vi "Load App.vi"(8 "error in (no error)":errorcluster, 11 "Status Notifier":refnum<notifier>) -> (0 "error out":errorcluster)   [LabVIEW 2012, in "Car Wash Controller.lvlib" / "Car Wash Controller.lvclass"]
doc: "Load the application into memory and start it running. The input notifier is used to send text to the splash screen to tell the user what stage the load process is in."
uses:
  Car Wash Controller.lvclass
  <vilib>/ActorFramework/Message Queue/Message Queue.lvclass/Message Queue.ctl
  <vilib>/ActorFramework/Actor/Actor.lvclass
  <vilib>/ActorFramework/Message Queue/Message Queue.lvclass
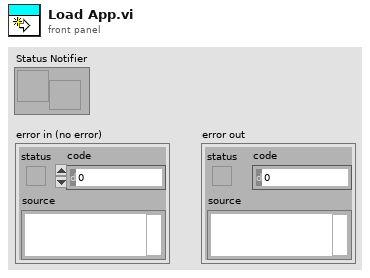
[diagram p1: front panel]
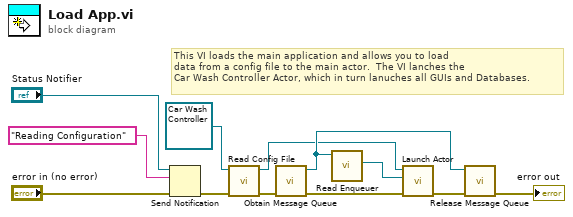
[diagram p0: block diagram]
diagram:
  # "This VI loads the main application and allows you to load\ndata from a config file to the main actor.  The VI lanches the\nCar Wash Controller Actor, which in turn lanuches all GUIs and Databases."
  n1 = Send Notification(notification="Reading Configuration", notifier="Status Notifier", error in (no error)="error in (no error)") -> (error out=w8:errorcluster)  [unwired: 1 out]
  n2 = call-dynamic "Read Config File.vi"("error in (no error)"=w8, "Car Wash CLA - Tom Fantasia in"=refnum<class "Car Wash Controller.lvclass"> refnum ("My Application.lvclass")) -> ("error out"=w4:errorcluster, "Car Wash CLA - Tom Fantasia out"=w1:refnum<class "Car Wash Controller.lvclass">)  [unwired: 8 in]
  n3 = call <vilib>:"Obtain Message Queue.vi"("error in (no error)"=w4) -> ("error out"=w3:errorcluster, "Message Queue"=w2:refnum<class "Message Queue.lvclass">)  [unwired: 9 in]
  n4 = call <vilib>:"Read Enqueuer.vi"("Message Queue"=w2) -> ("Message Enqueuer"=w7:refnum<class "Message Enqueuer.lvclass">)  [unwired: 10 in]
  n5 = call <vilib>:"Launch Actor.vi"("error in (no error)"=w3, "Actor-to-Caller Enqueuer"=w7, "Actor"=w1) -> ("error out"=w6:errorcluster)  [unwired: 7 in, 1 out]
  n6 = call <vilib>:"Release Message Queue.vi"("error in (no error)"=w6, "Message Queue"=w2) -> ("error out"=→"error out":errorcluster)  [unwired: 8 in, 1 out]
